vi "FPGA_CounterOpen & Configured.vi"(4 "IndexActiveHigh":bool=TRUE, 5 "External Reset":T1={"DevStatus"={"status"=FALSE, "code"=0, "source"=""}, "AnalogTriggerMode?"=FALSE, "DigitalMode"={"DIO Channel"=enum."Disabled"}, "AnalogTriggerMode"={"AnalogTriggerIndex"=enum."Trig 0", "OutputType"=enum."InWindow"}}, 6 "GTSDirThreshold":sgl, 7 "EdgeType":T5={"Master Mode"=enum."Edge Detection", "UpChannel"=enum."Disabled", "DownChannel"=enum."Disabled", "High/Up"=FALSE}, 8 "error in":errorcluster, 9 "DownSource":T1={"DevStatus"={"status"=FALSE, "code"=0, "source"=""}, "AnalogTriggerMode?"=FALSE, "DigitalMode"={"DIO Channel"=enum."Disabled"}, "AnalogTriggerMode"={"AnalogTriggerIndex"=enum."Trig 0", "OutputType"=enum."InWindow"}}, 10 "UpSource":T1={"DevStatus"={"status"=FALSE, "code"=0, "source"=""}, "AnalogTriggerMode?"=FALSE, "DigitalMode"={"DIO Channel"=enum."Disabled"}, "AnalogTriggerMode"={"AnalogTriggerIndex"=enum."Trig 0", "OutputType"=enum."InWindow"}}, 11 "CntIndex":T6=enum."Ctr 1") -> (0 "error out":errorcluster, 3 "Ctr Ref":T7={"DevStatus"={"status"=FALSE, "code"=0, "source"=""}, "CntIndex"=enum."Ctr 1"})   [LabVIEW 2017]
uses:
  <vilib>/Rock Robotics/SystemInterfaces/Counter/FPGA_CounterCtrDevRef.ctl
  <vilib>/Rock Robotics/SystemInterfaces/Counter/FPGA_CounterCtrSystemIndex.ctl
  <vilib>/Rock Robotics/SystemInterfaces/Counter/FPGA_CounterCtrEdgeDetectionType.ctl
  <vilib>/Rock Robotics/SystemInterfaces/CounterEncoderSourceConvertion/FPGA_CounterEncoderSourceConvertionLVSourceType.ctl
  <vilib>/Rock Robotics/SystemInterfaces/DIO/FPGA_DIODigitalSourceChannel.ctl
  <vilib>/Rock Robotics/SystemInterfaces/AnalogTrigger/FPGA_AnalogTriggerIndex.ctl
  <vilib>/Rock Robotics/SystemInterfaces/AnalogTrigger/FPGA_AnalogTriggerOutType.ctl
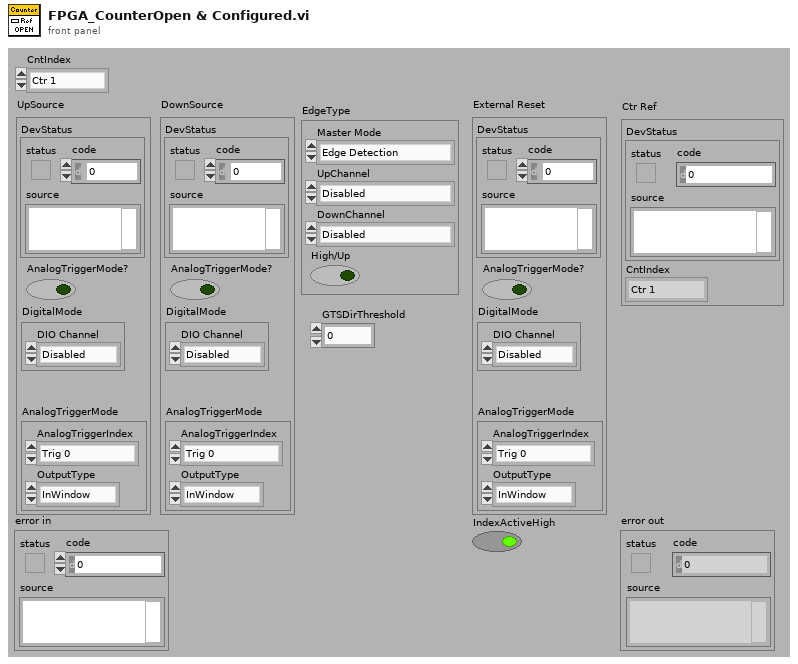
[diagram p1: front panel]
types:
  T1 = typedef "FPGA_CounterEncoderSourceConvertionLVSourceType.ctl" = cluster{"DevStatus":errorcluster, "AnalogTriggerMode?":bool, "DigitalMode":cluster{"DIO Channel":T2}, "AnalogTriggerMode":cluster{"AnalogTriggerIndex":T3, "OutputType":T4}}
  T2 = typedef "FPGA_DIODigitalSourceChannel.ctl" = enum8{"DIO 0", "DIO 1", "DIO 2", "DIO 3", "DIO 4", "DIO 5", "DIO 6", "DIO 7", "DIO 8", "DIO 9", "DIO MXP 0", "DIO MXP 1", "DIO MXP 2", "DIO MXP 3", "DIO MXP 4", "DIO MXP 5", "DIO MXP 6", "DIO MXP 7", "DIO MXP 8", "DIO MXP 9", "DIO MXP 10", "DIO MXP 11", "DIO MXP 12", "DIO MXP 13", "DIO MXP 14", "DIO MXP 15", "Disabled"}
  T3 = typedef "FPGA_AnalogTriggerIndex.ctl" = enum8{"Trig 0", "Trig 1", "Trig 2", "Trig 3", "Trig 4", "Trig 5", "Trig 6", "Trig 7", "Invalid"}
  T4 = typedef "FPGA_AnalogTriggerOutType.ctl" = enum16{"InWindow", "TriggerState", "Rising", "Falling"}
  T5 = typedef "FPGA_CounterCtrEdgeDetectionType.ctl" = cluster{"Master Mode":enum16{"Edge Detection", "Semi Period Mode", "Pulse Length Mode", "External Direction"}, "UpChannel":enum16{"Rising Edge", "Falling Edge", "Raising & Falling Edge", "Disabled"}, "DownChannel":enum16{"Rising Edge", "Falling Edge", "Raising & Falling Edge", "Disabled"}, "High/Up":bool}
  T6 = typedef "FPGA_CounterCtrSystemIndex.ctl" = enum8{"Ctr 0", "Ctr 1", "Ctr 2", "Ctr 3", "Ctr 4", "Ctr 5", "Ctr 6", "Ctr 7", "Invalid"}
  T7 = typedef "FPGA_CounterCtrDevRef.ctl" = cluster{"DevStatus":errorcluster, "CntIndex":T6}
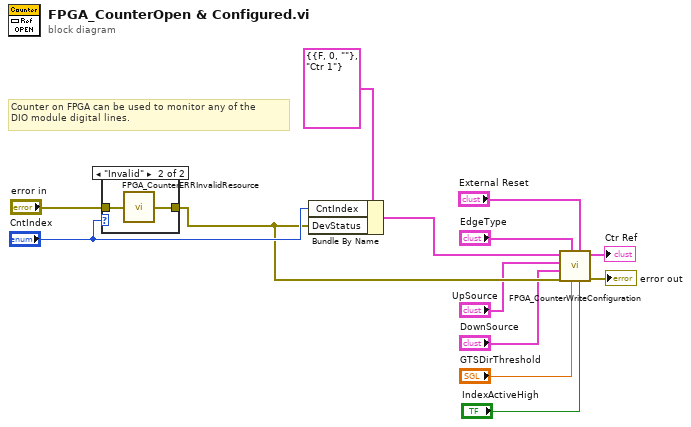
[diagram p0: block diagram]
diagram:
  # "Counter on FPGA can be used to monitor any of the \nDIO module digital lines."
  n1 = case shown="\"Invalid\"" "CntIndex" {
    tunnel: [w14 w16] -> w10
    tunnel: "error in" -> [w14 w15]
    frame Default {
    }
    frame "Invalid" {
      n2 = call <vilib>:"FPGA_CounterERRInvalidResource.vi"("error in (no error)"=w15) -> ("error out"=w16:errorcluster)
    }
  }
  n3 = Bundle By Name(cluster=T7 {"DevStatus"={"status"=FALSE, "code"=0, "source"=""}, "CntIndex"=enum."Ctr 1"} ("Ctr Ref"), "CntIndex"="CntIndex", "DevStatus"=w10) -> (w8:T7)
  n4 = call <vilib>:"FPGA_CounterWriteConfiguration.vi"("IndexActiveHigh"="IndexActiveHigh", "IndexSource"="External Reset", "GTSDirThreshold"="GTSDirThreshold", "EdgeType"="EdgeType", "error in (no error)"=w10, "DownSource"="DownSource", "UpSource"="UpSource", "Ctr Ref in"=w8) -> ("error out"=→"error out":errorcluster, "Ctr Ref out"=→"Ctr Ref":T7)  [unwired: 1 in, 1 out]
